vi "Theory Astar FPGA.vi"() -> ()   [LabVIEW 2014]
panel:
  out "XY Graph":T1(graph)
  out "Main y":i32[](array[numeric])
  out "Main X":i32[](array[numeric])
  out "Y Dest":i32
  out "X dest":i32
  in  "Destination Y":i16
  in  "Destination X":i16
  in  "Start Y":i16
  in  "Start X":i16
  in  "occupancy grid":bool[](array[boolean])=[FALSE, FALSE, FALSE, FALSE, FALSE, FALSE, FALSE, FALSE, FALSE, FALSE, FALSE, FALSE, FALSE, FALSE, FALSE, FALSE, FALSE, FALSE, FALSE, FALSE, FALSE, FALSE, FALSE, FALSE, FALSE, FALSE, FALSE, FALSE, FALSE, FALSE, FALSE, FALSE, FALSE, FALSE, FALSE, FALSE, FALSE, FALSE, FALSE, FALSE, FALSE, FALSE, FALSE, FALSE, FALSE, FALSE, FALSE, FALSE, FALSE, FALSE, FALSE, FALSE, FALSE, FALSE, FALSE, FALSE, FALSE, FALSE, FALSE, FALSE, FALSE, FALSE, FALSE, FALSE, FALSE, FALSE, FALSE, FALSE, FALSE, FALSE, FALSE, FALSE, FALSE, FALSE, FALSE, FALSE, FALSE, FALSE, FALSE, FALSE]
  # "x"
  # "y"
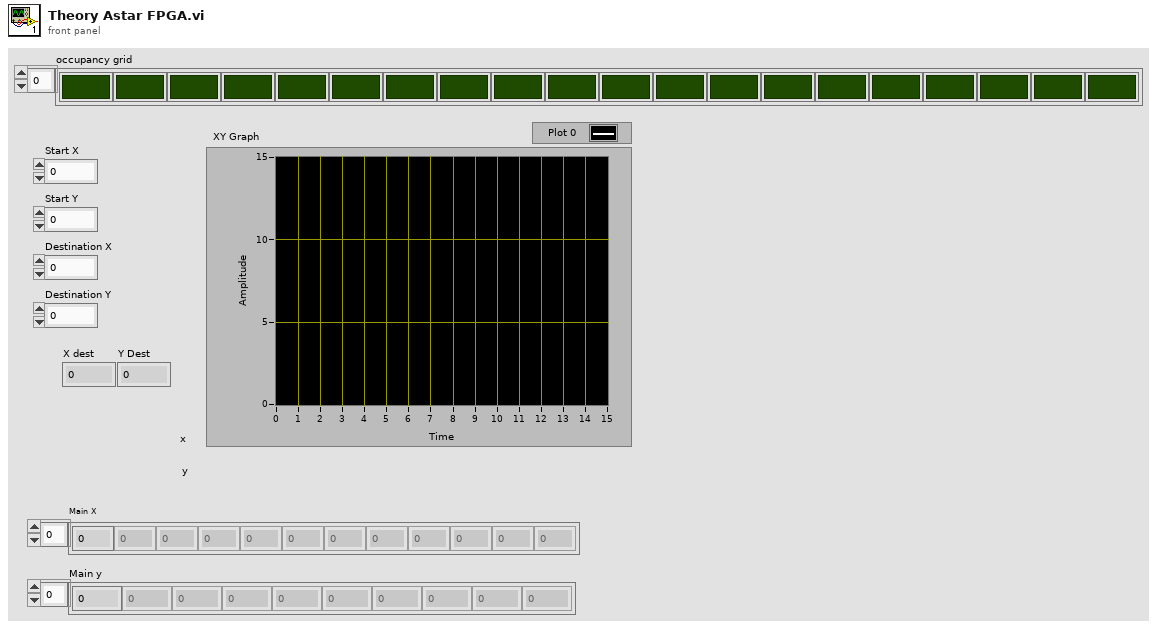
[diagram p1: front panel]
types:
  T1 = cluster{"dimension size":i32, "dimension size":i32}[]
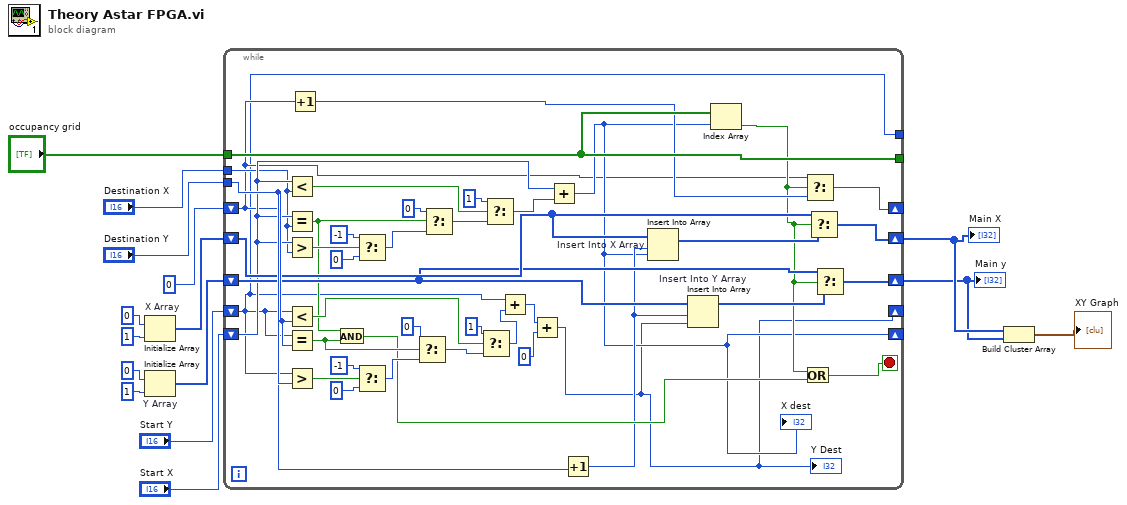
[diagram p0: block diagram]
diagram:
  n1 = Initialize Array "X Array"(0 ("dimension size"), 1 ("dimension size")) -> (w8:i32[])
  n2 = Initialize Array "Y Array"(0 ("dimension size"), 1 ("dimension size")) -> (w5:i32[])
  n3 = while {
    tunnel: "occupancy grid" -> [w36]
    tunnel: "Destination Y" -> [w57]
    tunnel: "Destination X" -> [w19]
    shift-right: [w21] -> _
    shift-left: "Start X" -> [w24]
    shift-right: [w20] -> _
    shift-left: "Start Y" -> [w16]
    shift-right: [w33] -> w2
    shift-left: w8 -> [w32]
    shift-right: [w34] -> _
    shift-left: 0 -> [w18]
    tunnel: [w36] -> _
    tunnel: [w16] -> _
    shift-right: [w31] -> w1
    shift-left: w5 -> [w30]
    stop <- w17 stop-if-true
    n4 = Less?(x=w24, y=w19) -> (x < y?=w49:bool)
    n5 = Equal?(x=w24, y=w19) -> (x = y?=w22:bool)
    n6 = Greater?(x=w24, y=w19) -> (0:w56:bool)
    n7 = Less?(x=w16, y=w57) -> (x < y?=w42:bool)
    n8 = Equal?(x=w16, y=w57) -> (x = y?=w38:bool)
    n9 = Greater?(x=w16, y=w57) -> (0:w41:bool)
    n10 = Increment(x=w18) -> (x+1=w35:i32)
    n11 = And(x=w22, y=w38) -> (x .and. y?=w37:bool)
    n12 = Select(t=-1, s=w56, f=0) -> (s? t:f=w52:i32)
    n13 = Select(t=-1, s=w41, f=0) -> (s? t:f=w45:i32)
    n14 = Select(t=0, s=w38, f=w45) -> (s? t:f=w43:i32)
    n15 = Select(t=0, s=w22, f=w52) -> (s? t:f=w50:i32)
    n16 = Select(t=1, s=w42, f=w43) -> (s? t:f=w39:i32)
    n17 = Select(t=1, s=w49, f=w50) -> (s? t:f=w40:i32)
    n18 = Add(x=w16, y=w39) -> (x+y=w26:i32)
    n19 = Add(x=w26, y=0) -> (x+y=w20:i32)
    "Y Dest" <- w20
    n20 = Add(x=w24, y=w40) -> (x+y=w21:i32)
    "X dest" <- w21
    n21 = Increment(x=w18) -> (x+1=w27:i32)
    n22 = Insert Into Array "Insert Into X Array"(array=w32, index=w27, new element=w21) -> (w29:i32[])
    n23 = Insert Into Array "Insert Into Y Array"(array=w30, index=w27, new element=w20) -> (w28:i32[])
    n24 = Index Array(array=w36, index=w21) -> (element=w23:bool)
    n25 = Or(x=w23, y=w37) -> (x .or. y?=w17:bool)
    n26 = Select(t=w18, s=w23, f=w35) -> (s? t:f=w34:i32)
    n27 = Select(t=w32, s=w23, f=w29) -> (s? t:f=w33:i32[])
    n28 = Select(t=w30, s=w23, f=w28) -> (s? t:f=w31:i32[])
  }
  "Main X" <- w2
  "Main y" <- w1
  n29 = Build Cluster Array(w2, w1) -> (→"XY Graph":T1)
